vi "Sent Get Public Events WFR.vi"(7 "Message Priority (Normal)":T2=enum."Normal", 8 "error in (no error)":errorcluster, 11 "Message Enqueuer":refnum<class "Message Enqueuer.lvclass">) -> (0 "error out":errorcluster, 2 "Reply":T1, 3 "Message Enqueuer out":refnum<class "Message Enqueuer.lvclass">)   [LabVIEW 2020, in "RPI.SenseHat.Actor.lvlib" / "Get Public Events Msg.lvclass"]
uses:
  Get Public Events Msg.lvclass
  <vilib>/ActorFramework/Message Enqueuer/Message Enqueuer.lvclass
  <vilib>/ActorFramework/Message Enqueuer/Message Priority.ctl
  C:/Program Files (x86)/National Instruments/LabVIEW 2020/vi.lib/ActorFramework/Reply Msg/Reply Msg.lvclass
  <vilib>/ActorFramework/Reply Msg/Reply Msg.lvclass/Reply Msg.ctl
  <vilib>/ActorFramework/Message Enqueuer/Message Enqueuer.lvclass/Message Enqueuer.ctl
  <vilib>/ActorFramework/Message Enqueuer/Enqueue.vi
  <vilib>/ActorFramework/Reply Msg/Reply Msg.lvclass
  C:/Program Files (x86)/National Instruments/LabVIEW 2020/vi.lib/ActorFramework/Message/Message.lvclass
  <vilib>/ActorFramework/Message Priority Queue/Priority Enqueue.vi
  RPI.SenseHat.Joystick/TypeDefs/Joystick.ctl
  RPI.SenseHat.Joystick/RPI.SenseHat.Joystick.lvlib
  RPI.SenseHat.Actor/Public Events.ctl
  RPI.SenseHat.Actor/RPI.SenseHat.Actor.lvclass
  Z:/Code/Git/WC/RPI.SenseHat/src/RPI.SenseHat.Actor/RPI.SenseHat.Actor Messages/Get Public Events Msg/Get Public Events Msg.lvclass
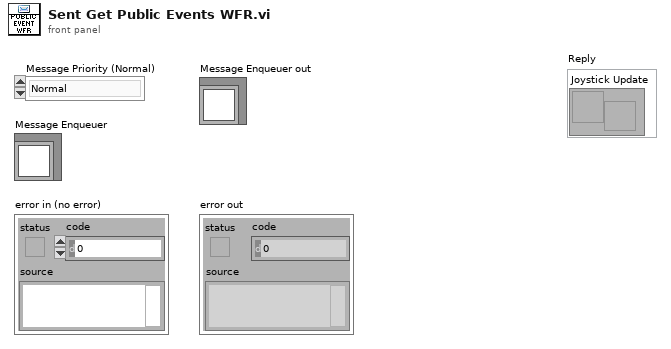
[diagram p1: front panel]
types:
  T1 = typedef "RPI.SenseHat.Actor.lvlib/RPI.SenseHat.Actor.lvclass/Public Events.ctl" = cluster{"Joystick Update":refnum<user-event>}
  T2 = typedef "Actor Framework.lvlib/Message Enqueuer.lvclass/Message Priority.ctl" = enum16{"Low", "Normal", "High"}
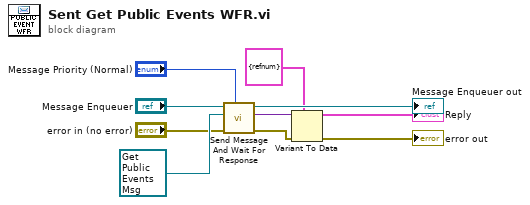
[diagram p0: block diagram]
diagram:
  n1 = call <vilib>:"Send Message And Wait For Response.vi"("Message Priority (Normal)"="Message Priority (Normal)", "error in (no error)"="error in (no error)", "Original Message"=refnum<class "Get Public Events Msg.lvclass"> refnum ("RPI.SenseHat.Actor.lvlib:Get Public Events Msg.lvclass"), "Message Enqueuer in"="Message Enqueuer") -> ("error out"=w4:errorcluster, "Reply"=w5:variant, "Message Enqueuer out"=→"Message Enqueuer out":refnum<class "Message Enqueuer.lvclass">)  [unwired: 4 in, 1 out]
  n2 = Variant To Data(error in=w4, type=T1 {"Joystick Update"=refnum}, Variant=w5) -> (data=→"Reply":T1, error out=→"error out":errorcluster)
